vi "set_speed_params.vi"(6 "pixel-dwell time":dbl[unit]=-1.0, 8 "error in (no error)":errorcluster, 9 "line-scan time":dbl[unit]=-1.0, 10 "frame rate":dbl[unit]=-1.0, 11 "ImagingModeDL090130Frame in":refnum<class "ImagingModeDL090130Frame.lvclass">) -> (0 "error out":errorcluster, 3 "ImagingModeDL090130Frame out":refnum<class "ImagingModeDL090130Frame.lvclass">)   [LabVIEW 2010, in "ImagingModeDL090130Frame.lvclass"]
uses:
  ImagingModeDL090130Frame.lvclass
  ImagingModeDL090130Frame.lvclass/ImagingModeDL090130Frame.ctl
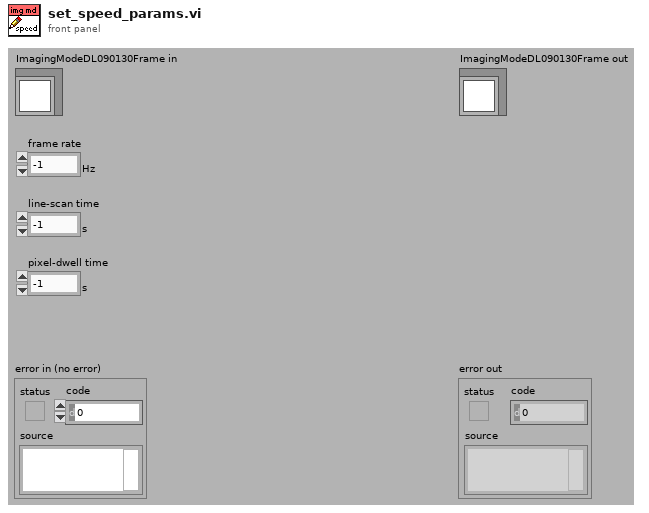
[diagram p1: front panel]
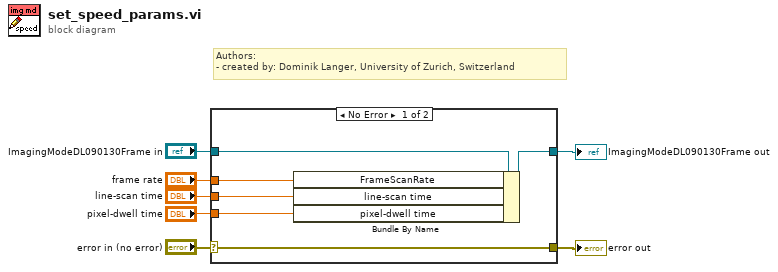
[diagram p0: block diagram]
diagram:
  # "Authors: \n- created by: Dominik Langer, University of Zurich, Switzerland"
  n1 = case shown="No Error" "error in (no error)" {
    selector: "error in (no error)" -> [w13 w15]
    tunnel: [w13 w15] -> w6
    tunnel: [w8 w14] -> w4
    tunnel: "ImagingModeDL090130Frame in" -> [w9 w14]
    tunnel: "frame rate" -> [w12 _]
    tunnel: "line-scan time" -> [w11 _]
    tunnel: "pixel-dwell time" -> [w10 _]
    frame No Error {
      n2 = Bundle By Name(cluster=w9, "FrameScanRate"=w12, "line-scan time"=w11, "pixel-dwell time"=w10) -> (w8:refnum<class "ImagingModeDL090130Frame.lvclass">)
    }
    frame Error {
    }
  }
  "error out" <- w6
  "ImagingModeDL090130Frame out" <- w4
